vi "Name FIFO.vi"(10 "Values for Naming":T1={"Bus Number"=1, "Device Number"=1, "Channel Number"=1} {"Channel Number" min=1 step=1; "Device Number" min=1 step=1; "Bus Number" min=1 step=1}, 11 "Current Loop Iteration Even":bool) -> (3 "FIFO Name":string)   [LabVIEW 2014, in "Initialization and IO Node Scripting.lvlib"]
uses:
  Initialization and IO Node Scripting.lvlib
  State Machine/Controls/Values for Naming.ctl
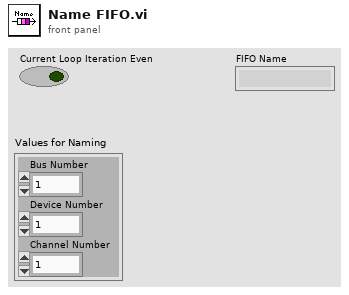
[diagram p1: front panel]
types:
  T1 = typedef "Initialization and IO Node Scripting.lvlib/Values for Naming.ctl" = cluster{"Bus Number":i32, "Device Number":i32, "Channel Number":i32}
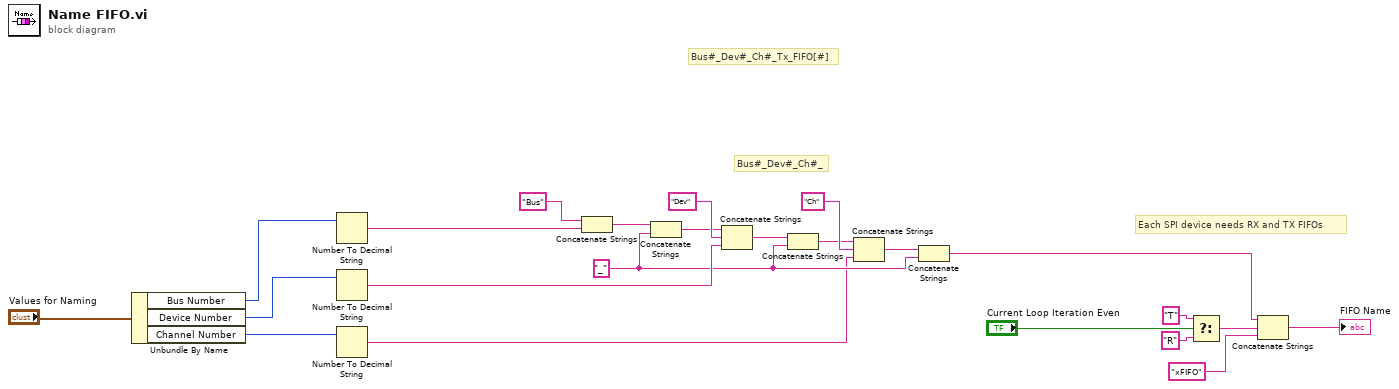
[diagram p0: block diagram]
diagram:
  w15 = "_" ("string")
  # "Bus#_Dev#_Ch#_"
  # "Bus#_Dev#_Ch#_Tx_FIFO[#]"
  # "Each SPI device needs RX and TX FIFOs"
  n1 = Unbundle By Name("Values for Naming") -> ("Bus Number"=w6:i32, "Device Number"=w1:i32, "Channel Number"=w2:i32)
  n2 = Number To Decimal String(number=w6) -> (decimal integer string=w16:string)  [unwired: 1 in]
  n3 = Number To Decimal String(number=w1) -> (decimal integer string=w17:string)  [unwired: 1 in]
  n4 = Number To Decimal String(number=w2) -> (decimal integer string=w3:string)  [unwired: 1 in]
  n5 = Concatenate Strings("Bus" ("string"), w16) -> (w8:string)
  n6 = Concatenate Strings(w8, w15) -> (w9:string)
  n7 = Concatenate Strings(w9, "Dev" ("string"), w17) -> (w11:string)
  n8 = Concatenate Strings(w11, w15) -> (w12:string)
  n9 = Concatenate Strings(w12, "Ch" ("string"), w3) -> (w14:string)
  n10 = Concatenate Strings(w14, w15) -> (w4:string)
  n11 = Select(t="T" ("string"), s="Current Loop Iteration Even", f="R" ("string")) -> (s? t:f=w22:string)
  n12 = Concatenate Strings(w4, w22, "xFIFO" ("string")) -> (→"FIFO Name":string)
